vi "IntakeForTime.vi"() -> ()   [LabVIEW 2018]
uses:
  Framework/Robot Global Data.vi
panel:
  in  "NoWait":bool
  in  "Speed":dbl=1.0
  in  "Time":dbl=3.0
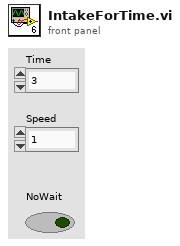
[diagram p1: front panel]
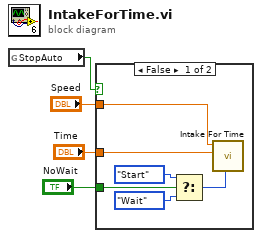
[diagram p0: block diagram]
diagram:
  n1 = global read "Robot Global Data.vi" "StopAuto"() -> (w4:bool)
  n2 = case shown="False" w4 {
    tunnel: "Time" -> [w9 _]
    tunnel: "Speed" -> [w10 _]
    tunnel: "NoWait" -> [w8 _]
    frame False {
      n3 = Select(t=enum16{"Start", "Wait"}."Start" ("Synchronization"), s=w8, f=enum16{"Start", "Wait"}."Wait" ("Synchronization")) -> (s? t:f=w5:enum16{"Start", "Wait"})
      n4 = call "Intake For Time.vi"("Synchronization"=w5, "Duration (s)"=w9, "Speed"=w10) -> ()  [unwired: 8 in, 1 out]
    }
    frame True {
    }
  }
